vi "Func Head-Foot replacer.vi"(5 "Function in":string, 11 "error in (no error)":errorcluster) -> (4 "No. of braces":i32, 6 "Function in Out":string, 15 "error out":errorcluster)   [LabVIEW 2014]
doc: "This VI replace \"(\" and \")\" with \"SOP\" and \"EOP\" from function math.\n\nDesigned by HB\nhaba@dtu.dk"
panel:
  out "flag":i32
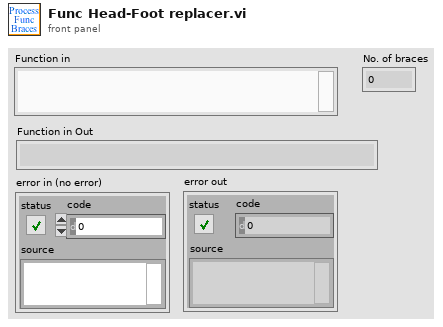
[diagram p1: front panel]
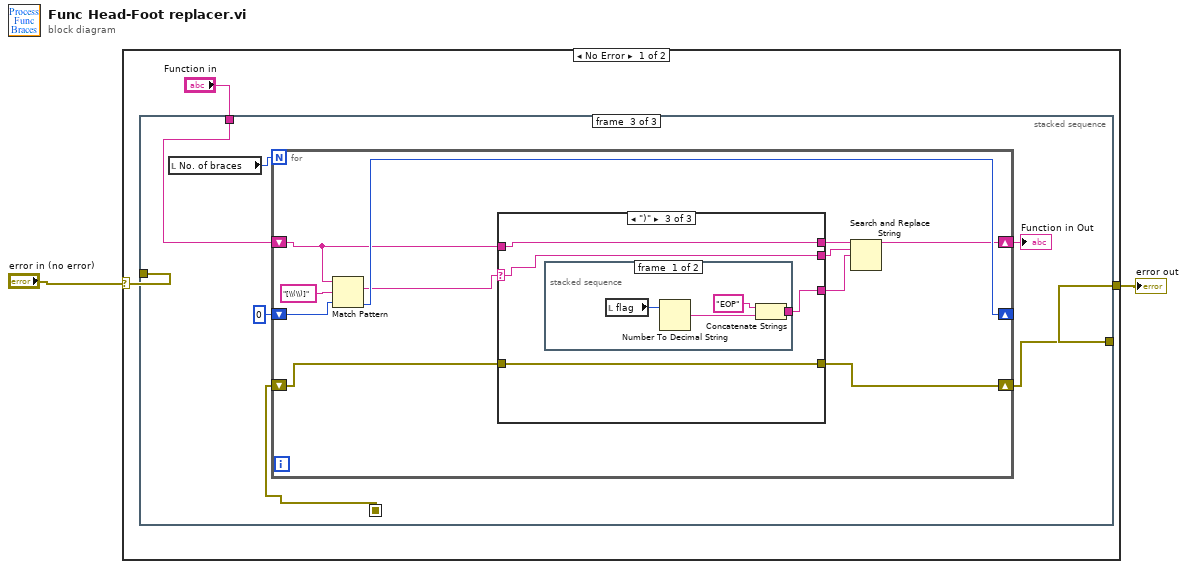
[diagram p0: block diagram]
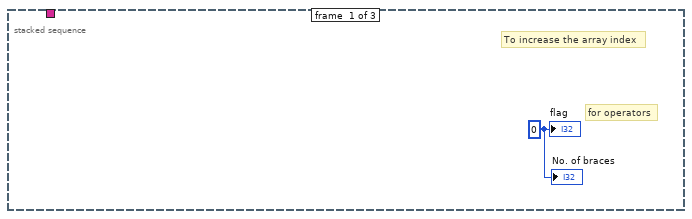
[diagram p2: hidden frame]
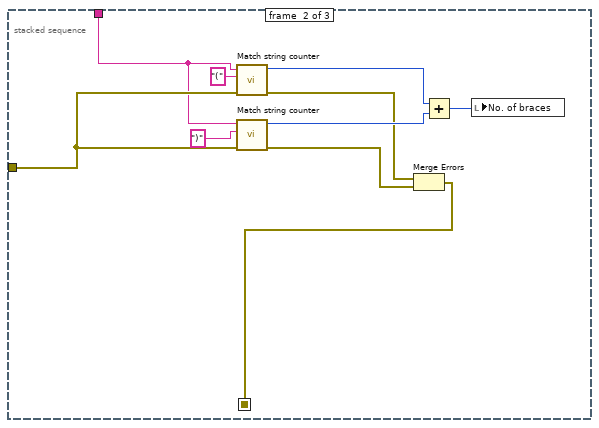
[diagram p3: hidden frame]
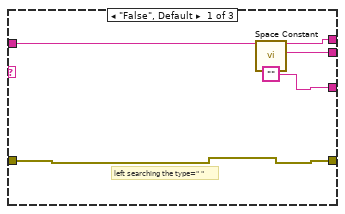
[diagram p4: hidden frame]
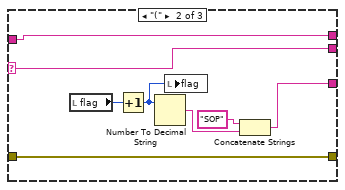
[diagram p5: hidden frame]
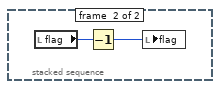
[diagram p6: hidden frame]
diagram:
  n1 = case shown="No Error" "error in (no error)" {
    selector: "error in (no error)" -> [w3 w56]
    tunnel: [w4 w56] -> w2
    frame No Error {
      n2 = stacked-sequence {
        seq-local: [_ w9 _] -> [_ _ w18]
        tunnel: "Function in" -> [_ w7 w21]
        tunnel: w3 -> [_ w12 _]
        tunnel: [_ _ w20] -> w4
        frame #0 {
          w6 = 0 ("App_Cnt")
          # "To increase the array index"
          # "for operators"
          "flag" <- w6
          "No. of braces" <- w6
        }
        frame #1 {
          n3 = call "Match string counter.vi"("error in (no error)"=w12, "Match String"="(", "Input string"=w7) -> ("error out"=w11:errorcluster, "Count"=w15:i32)  [unwired: 7 in]
          n4 = call "Match string counter.vi"("error in (no error)"=w12, "Match String"=")", "Input string"=w7) -> ("error out"=w10:errorcluster, "Count"=w14:i32)  [unwired: 7 in]
          n5 = Merge Errors(w11, w10) -> (w9:errorcluster)
          n6 = Add(x=w15, y=w14) -> (x+y=w13:i32)
          n7 = local write "No. of braces"(w13) -> ()
        }
        frame #2 {
          n8 = local read "No. of braces"() -> (w19:i32)
          n9 = for {
            N: w19 -> [_]
            shift-right: [w32] -> _
            shift-left: 0 ("offset past match") -> [w31]
            shift-right: [w29] -> w20
            shift-left: w18 -> [w30]
            shift-right: [w26] -> w17
            shift-left: w21 -> [w27]
            n10 = Match Pattern(string=w27, regular expression="[\\(\\)]" ("Match String"), offset (0)=w31) -> (match substring=w28:string, offset past match=w32:i32)  [unwired: 2 out]
            n11 = case shown="\")\"" w28 {
              selector: w28 -> [_ w38 w46]
              tunnel: ["" ("string") w45 w49] -> w23
              tunnel: w30 -> [w34 w40 w48]
              tunnel: [w34 w40 w48] -> w29
              tunnel: w27 -> [w37 w39 w47]
              tunnel: [w37 w39 w47] -> w25
              tunnel: [w36 w38 w46] -> w24
              frame "False", Default {
                # "left searching the type=\" \""
                n12 = call <vilib>:"Space Constant.vi"() -> ("String"=w36:string)
              }
              frame "(" {
                n13 = local read "flag"() -> (w42:i32)
                n14 = Increment(x=w42) -> (x+1=w43:i32)
                n15 = Number To Decimal String(number=w43) -> (decimal integer string=w44:string)  [unwired: 1 in]
                n16 = local write "flag"(w43) -> ()
                n17 = Concatenate Strings("SOP", w44) -> (w45:string)
              }
              frame ")" {
                n18 = stacked-sequence {
                  tunnel: [w52 _] -> w49
                  frame #0 {
                    n19 = local read "flag"() -> (w50:i32)
                    n20 = Number To Decimal String(number=w50) -> (decimal integer string=w51:string)  [unwired: 1 in]
                    n21 = Concatenate Strings("EOP", w51) -> (w52:string)
                  }
                  frame #1 {
                    n22 = local read "flag"() -> (w54:i32)
                    n23 = Decrement(x=w54) -> (x-1=w55:i32)
                    n24 = local write "flag"(w55) -> ()
                  }
                }
              }
            }
            n25 = Search and Replace String(input string=w25, search string=w24, replace string=w23) -> (result string=w26:string)  [unwired: 5 in, 3 out]
          }
          "Function in Out" <- w17
        }
      }
    }
    frame Error {
    }
  }
  "error out" <- w2
